vi "Edit Config.vi"(8 "error in (no error)":errorcluster, 11 "NI Analog in":refnum<class "Num Array.lvclass">) -> (0 "error out":errorcluster, 3 "NI Analog out":refnum<class "Num Array.lvclass">)   [LabVIEW 2018, in "Num Array.lvclass"]
doc: "NI Analog Out.lvclass:Edit Config.vi\n\nThis VI is used to edit the NI Analog Out configuration parameters.\n\nInstrument Communication Module Version 1.0\nOctober, 2020 Original Code Consulting Davita Bird\n www.originalcode.com"
uses:
  Num Array.lvclass
  NI AO Type Def.ctl
  Controls/ICM Class Editor State.ctl
  Controls/ICM Editor Command.ctl
  Num Array.lvclass/Num Array.ctl
panel:
  out "Device Table":string[][](table)
  in  "Num Array Config":T1
  in  "Flash Save":bool
  in  "Save":bool
  in  "Revert":bool
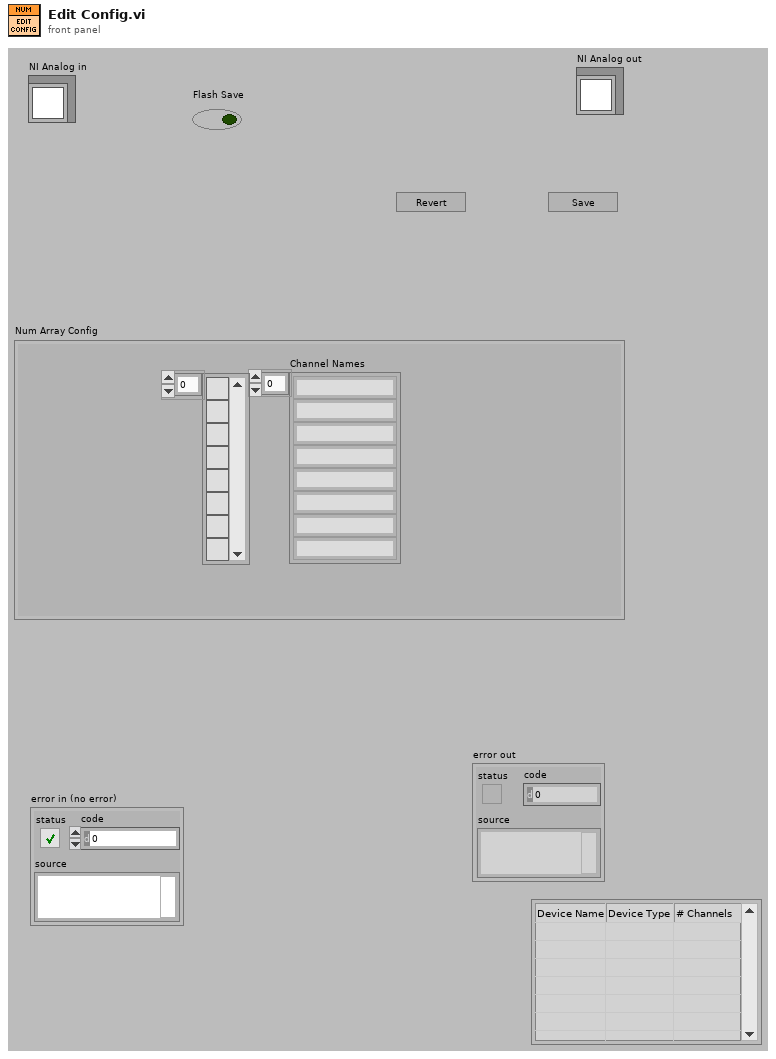
[diagram p1: front panel]
types:
  T1 = typedef "NI AO Type Def.ctl" = cluster{"Channel Names":string[], "Enabled":bool[]}
  T2 = typedef "ICM Editor Command.ctl" = enum16{"No-op", "Exit"}
  T3 = typedef "ICM Class Editor State.ctl" = enum16{"Init", "Wait", "Write", "Read", "Display", "Set Flashing", "Error", "Stop"}
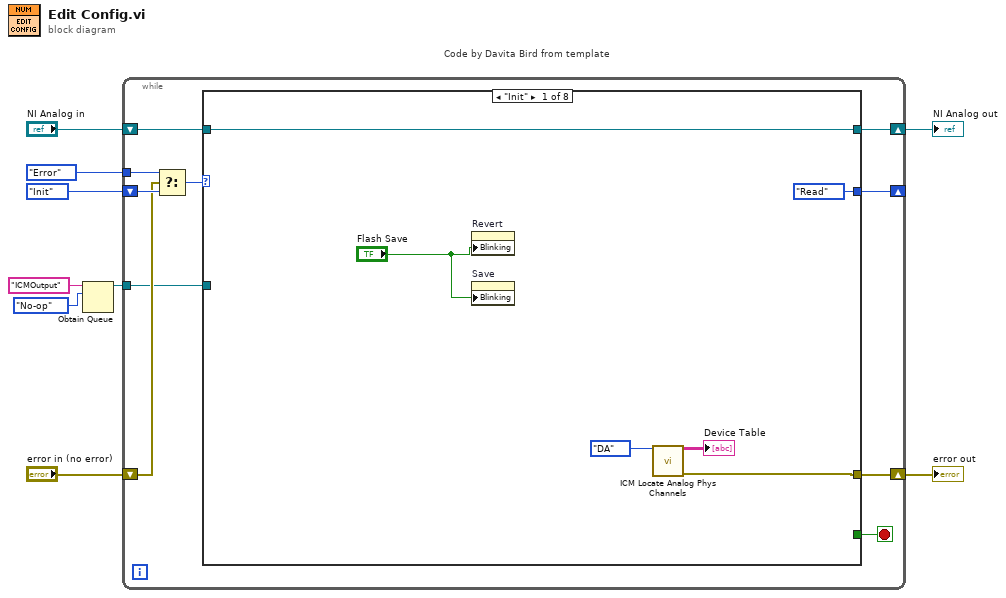
[diagram p0: block diagram]
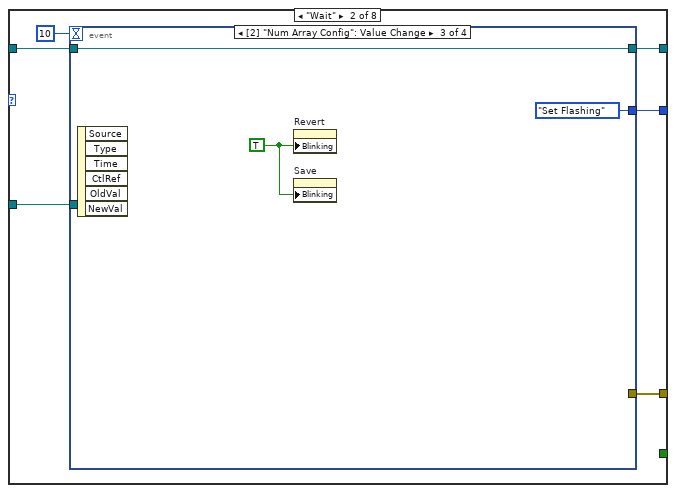
[diagram p2: hidden frame]
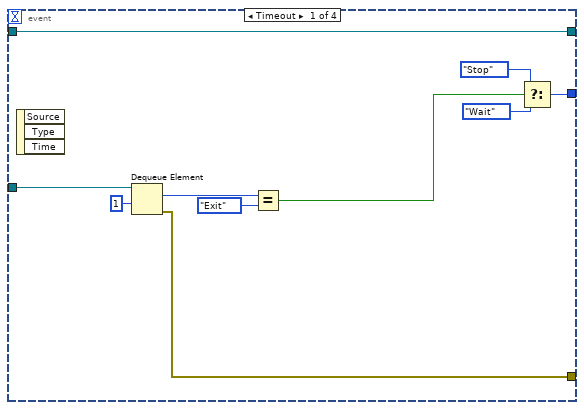
[diagram p3: hidden frame]
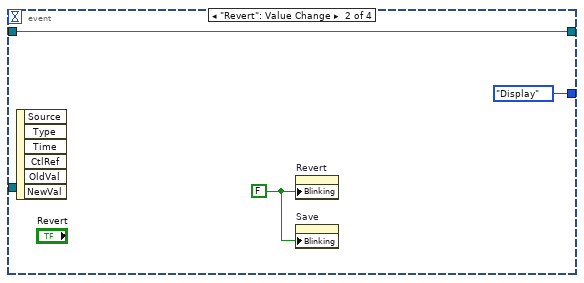
[diagram p4: hidden frame]
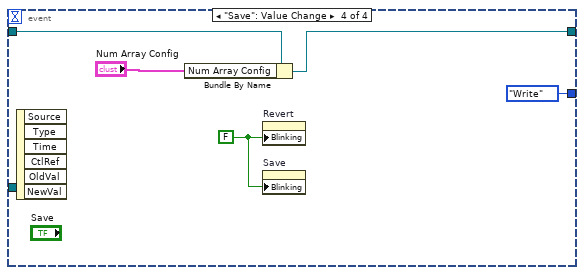
[diagram p5: hidden frame]
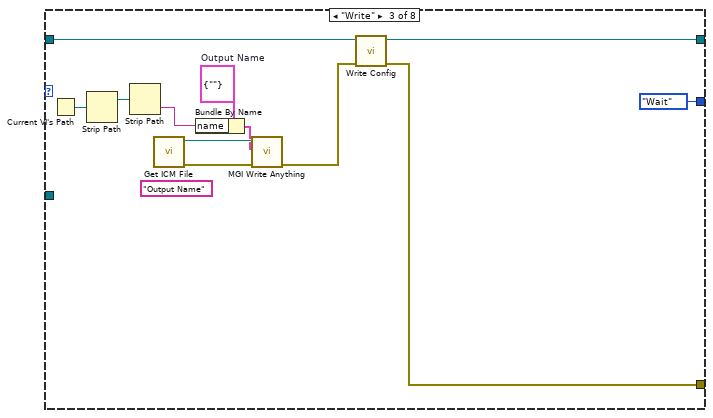
[diagram p6: hidden frame]
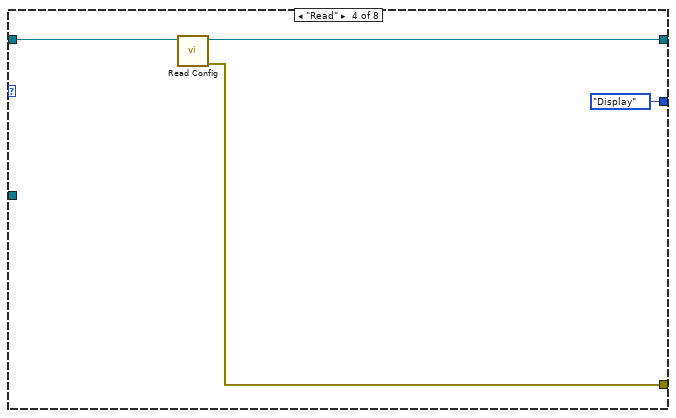
[diagram p7: hidden frame]
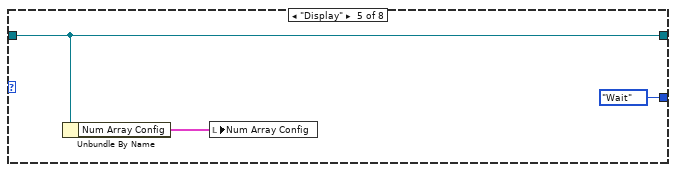
[diagram p8: hidden frame]
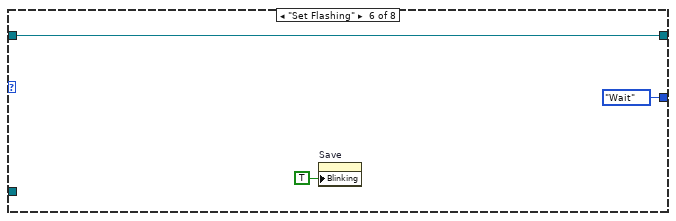
[diagram p9: hidden frame]
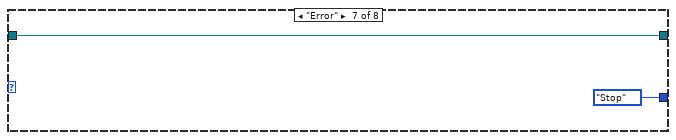
[diagram p10: hidden frame]
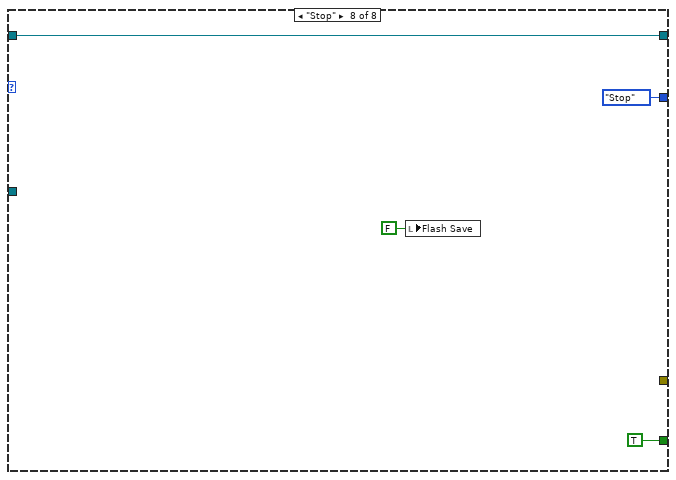
[diagram p11: hidden frame]
diagram:
  n1 = Obtain Queue(name (unnamed)="ICMOutput", element data type=ICM_Editor_Command."No-op" ("Editor Command")) -> (queue out=w1:refnum<queue>)  [unwired: 3 in, 2 out]
  n2 = while "Code by Davita Bird from template" {
    shift-right: [w19] -> w8
    shift-left: "NI Analog in" -> [w18]
    shift-right: [w12] -> _
    shift-left: ICM_Class_Editor_State."Init" ("Config State") -> [w16]
    shift-right: [w11] -> w6
    shift-left: "error in (no error)" -> [w14]
    tunnel: ICM_Class_Editor_State."Error" ("Config State") -> [w13]
    tunnel: w1 -> [w10]
    stop <- w17 stop-if-true
    n3 = Select(t=w13, s=w14, f=w16) -> (s? t:f=w15:T3)
    n4 = case shown="\"Init\"" w15 {
      tunnel: [w24 w29 w62 w66 w71 w74 w76 w80] -> w19
      tunnel: w18 -> [w24 w28 w63 w68 w71 w74 w76 w80]
      tunnel: [_ _ _ _ _ _ _ TRUE] -> w17
      tunnel: [ICM_Class_Editor_State."Read" ("Config State") w30 ICM_Class_Editor_State."Wait" ("Config State") ICM_Class_Editor_State."Display" ("Config State") ICM_Class_Editor_State."Wait" ("Config State") ICM_Class_Editor_State."Wait" ("Config State") ICM_Class_Editor_State."Stop" ("Config State") ICM_Class_Editor_State."Stop" ("Config State")] -> w12
      tunnel: [w20 w26 w61 w67 _ _ _ _] -> w11
      tunnel: w10 -> [_ w27 _ _ _ _ _ _]
      frame "Init" {
        n5 = property on="Revert" class="Bool"("Blinking"="Flash Save") -> ()  [unwired: 2 in, 2 out]
        n6 = property on="Save" class="Bool"("Blinking"="Flash Save") -> ()  [unwired: 2 in, 2 out]
        n7 = call "ICM Locate Analog Phys Channels.vi"("Channel Type"=enum16{"AD SE", "AD Diff", "DA"}."DA") -> ("Table"=→"Device Table":string[][], "error out"=w20:errorcluster)  [unwired: 13 in]
      }
      frame "Wait" {
        n8 = event shown="[2] \"Num Array Config\": Value Change" {
          selector: _ -> [_ _ _ _]
          dyn-events: _ -> [_ _ _ _]
          timeout: 10 -> [_ _ _ _]
          tunnel: [w38 ICM_Class_Editor_State."Display" ("Config State") ICM_Class_Editor_State."Set Flashing" ("Config State") ICM_Class_Editor_State."Write" ("Config State")] -> w30
          tunnel: [w41 w43 w47 w50] -> w29
          tunnel: w28 -> [w41 w43 w47 w51]
          tunnel: w27 -> [w40 _ _ _]
          tunnel: [w32 _ _ _] -> w26
          event Timeout {
            n9 = event-data() -> ()  [unwired: 1 in, 3 out]
            n10 = Dequeue Element(queue=w40, timeout in ms (-1)=1) -> (element=w37:T2, error out=w32:errorcluster)  [unwired: 1 in, 2 out]
            n11 = Equal?(x=w37, y=ICM_Editor_Command."Exit") -> (x = y?=w35:bool)
            n12 = Select(t=ICM_Class_Editor_State."Stop" ("Config State"), s=w35, f=ICM_Class_Editor_State."Wait" ("Config State")) -> (s? t:f=w38:T3)
          }
          event "Revert": Value Change {
            w42 = FALSE ("Blinking")
            n13 = event-data() -> ()  [unwired: 1 in, 6 out]
            n14 = property on="Revert" class="Bool"("Blinking"=w42) -> ()  [unwired: 2 in, 2 out]
            n15 = property on="Save" class="Bool"("Blinking"=w42) -> ()  [unwired: 2 in, 2 out]
          }
          event Value Change {
            w45 = TRUE ("Blinking")
            n16 = event-data() -> ()  [unwired: 1 in, 6 out]
            n17 = property on="Revert" class="Bool"("Blinking"=w45) -> ()  [unwired: 2 in, 2 out]
            n18 = property on="Save" class="Bool"("Blinking"=w45) -> ()  [unwired: 2 in, 2 out]
          }
          event "Save": Value Change {
            w49 = FALSE ("Blinking")
            n19 = event-data() -> ()  [unwired: 1 in, 6 out]
            n20 = Bundle By Name(cluster=w51, "Num Array Config"="Num Array Config") -> (w50:refnum<class "Num Array.lvclass">)
            n21 = property on="Revert" class="Bool"("Blinking"=w49) -> ()  [unwired: 2 in, 2 out]
            n22 = property on="Save" class="Bool"("Blinking"=w49) -> ()  [unwired: 2 in, 2 out]
          }
        }
      }
      frame "Write" {
        w55 = cluster{"name":string} {"name"=""}  # Output Name
        (unwired) "Output Name" ("Section Name (Name of \"Anything\")")
        n23 = Current VI's Path() -> (path=w60:path)
        n24 = Strip Path(path=w60) -> (stripped path=w59:path)  [unwired: 1 out]
        n25 = Strip Path(path=w59) -> (name=w54:string)  [unwired: 1 out]
        n26 = call "Get ICM File.vi"() -> ("error out"=w57:errorcluster, "ICM File"=w58:path)  [unwired: 10 in]
        n27 = Bundle By Name(cluster=w55, "name"=w54) -> (w53:cluster{"name":string})
        n28 = call <userlib>:"MGI Write Anything.vi"("Error In"=w57, "Anything"=w53, "Path (dialog)"=w58) -> ("Error Out"=w56:errorcluster)  [unwired: 6 in, 2 out]
        n29 = call-dynamic "Write Config.vi"("error in (no error)"=w56, "Num Array in"=w63) -> ("error out"=w61:errorcluster, "Num Array out"=w62:refnum<class "Num Array.lvclass">)  [unwired: 8 in]
      }
      frame "Read" {
        n30 = call-dynamic "Read Config.vi"("Num Array in"=w68) -> ("error out"=w67:errorcluster, "Num Array out"=w66:refnum<class "Num Array.lvclass">)  [unwired: 9 in]
      }
      frame "Display" {
        n31 = Unbundle By Name(w71) -> ("Num Array Config"=w70:T1)
        n32 = local write "Num Array Config"(w70) -> ()
      }
      frame "Set Flashing" {
        n33 = property on="Save" class="Bool"("Blinking"=TRUE) -> ()  [unwired: 2 in, 2 out]
      }
      frame "Error" {
      }
      frame "Stop" {
        n34 = local write "Flash Save"(FALSE ("Flash Save")) -> ()
      }
    }
  }
  "error out" <- w6
  "NI Analog out" <- w8
